vi "provide_note_book_info.vi"(8 "error in (no error)":errorcluster, 10 "notebook string in":string, 11 "TrajectoryAK101022Resonance in":refnum<class "TrajectoryAK101022Resonance.lvclass">) -> (0 "error out":errorcluster, 2 "notebook string out":string, 3 "TrajectoryAK101022Resonance out":refnum<class "TrajectoryAK101022Resonance.lvclass">)   [LabVIEW 2010, in "TrajectoryAK101022Resonance.lvclass"]
uses:
  TrajectoryAK101022Resonance.lvclass
  TrajectoryAK101022Resonance.lvclass/TrajectoryAK101022Resonance.ctl
  TrajectoryMG100122GenericFPGA/TrajectoryMG100122GenericFPGA/TrajectoryMG100122GenericFPGA.lvclass
  common/classes/ErrorController/ErrorController/class_data.vi
  common/classes/ErrorController/ErrorController/ErrorController.lvclass
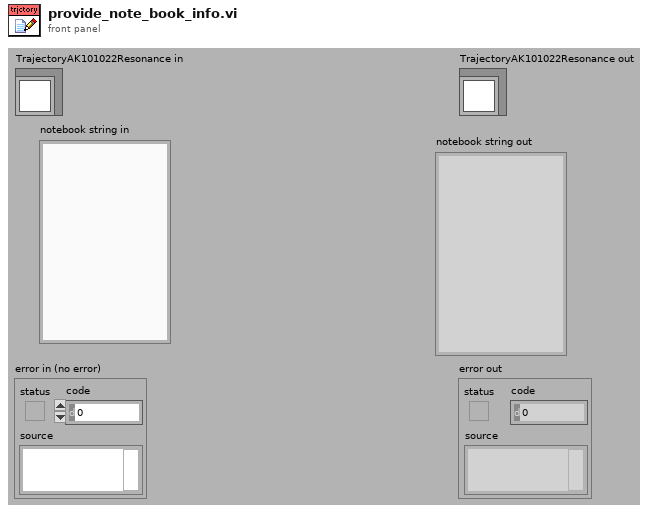
[diagram p1: front panel]
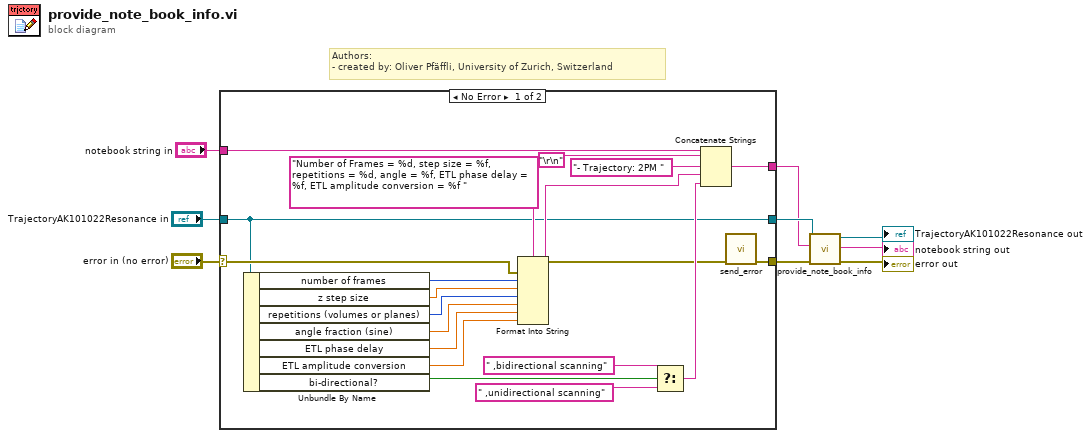
[diagram p0: block diagram]
diagram:
  # "Authors: \n- created by: Oliver Pfäffli, University of Zurich, Switzerland"
  n1 = case shown="No Error" "error in (no error)" {
    selector: "error in (no error)" -> [w20 w32]
    tunnel: [w11 w32] -> w5
    tunnel: "TrajectoryAK101022Resonance in" -> [w10 w31]
    tunnel: "notebook string in" -> [w29 w30]
    tunnel: [w26 w30] -> w2
    tunnel: [w10 w31] -> w4
    frame No Error {
      n2 = Unbundle By Name(w10) -> ("number of frames"=w19:i32, "z step size"=w18:dbl[unit], "repetitions (volumes or planes)"=w17:i32, "angle fraction (sine)"=w16:dbl, "ETL phase delay"=w15:dbl[unit], "ETL amplitude conversion"=w14:dbl[unit], "bi-directional?"=w13:bool)
      n3 = Format Into String(format string="Number of Frames = %d, step size = %f, repetitions = %d, angle = %f, ETL phase delay = %f, ETL amplitude conversion = %f ", error in=w20, w19, w18, w17, w16, w15, w14) -> (resulting string=w24:string, error out=w12:errorcluster)  [unwired: 1 in]
      n4 = Select(t=" ,bidirectional scanning" ("initial string"), s=w13, f=" ,unidirectional scanning" ("initial string")) -> (s? t:f=w21:string)
      n5 = Concatenate Strings(w29, "\r\n", "- Trajectory: 2PM " ("string"), w24, w21) -> (w26:string)
      n6 = call "send_error.vi"("error in (no error)"=w12) -> ("error out"=w11:errorcluster)  [unwired: 10 in]
    }
    frame Error {
    }
  }
  n7 = call-parent "provide_note_book_info.vi"("error in (no error)"=w5, "notebook string in"=w2, "GenericPlugin in"=w4) -> ("error out"=→"error out":errorcluster, "notebook string out"=→"notebook string out":string, "GenericPlugin out"=→"TrajectoryAK101022Resonance out":refnum<class "TrajectoryAK101022Resonance.lvclass">)  [unwired: 6 in]
